vi "CRYTable Empty Ignore.vi"(11 "Table In":string[][](array[string])) -> (3 "Table Out":string[][](array[string]))   [LabVIEW 2013]
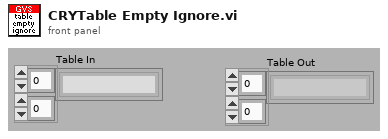
[diagram p1: front panel]
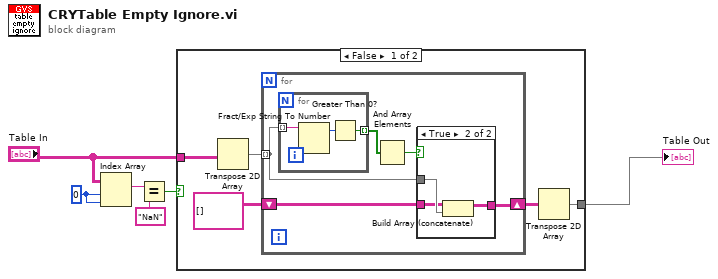
[diagram p0: block diagram]
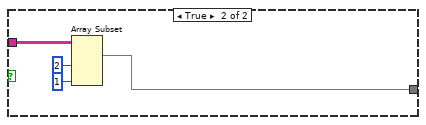
[diagram p3: hidden frame]
diagram:
  w6 = 0 ("Index")
  n1 = Index Array(array="Table In", index (row)=w6, index (col)=w6) -> (element=w5:string)
  n2 = Equal?(x=w5, y="NaN") -> (x = y?=w3:bool)
  n3 = case shown="False" w3 {
    tunnel: "Table In" -> [w11 w25]
    tunnel: [w7 w24] -> w1
    frame False {
      n4 = Transpose 2D Array(2D array=w11) -> (transposed array=w10:string[][])
      n5 = for {
        shift-right: [w16] -> w8
        shift-left: string[][] [] -> [w15]
        tunnel: w10 -> [w13] mode=indexing
        n6 = for {
          tunnel: w13 -> [w19] mode=indexing
          tunnel: [w17] -> w12 mode=indexing
          n7 = Fract/Exp String To Number(string=w19) -> (offset past number=w18:i32)  [unwired: 4 out]
          n8 = Greater Than 0?(x=w18) -> (x > 0?=w17:bool)
        }
        n9 = And Array Elements(Boolean array=w12) -> (logical AND=w14:bool)
        n10 = case shown="True" w14 {
          tunnel: w13 -> [_ w23]
          tunnel: [w20 w22] -> w16
          tunnel: w15 -> [w20 w21]
          frame False {
          }
          frame True {
            n11 = Build Array (concatenate)(w21, w23) -> (w22:string[][])
          }
        }
      }
      n12 = Transpose 2D Array(2D array=w8) -> (transposed array=w7:string[][])
    }
    frame True {
      n13 = Array Subset(array=w25, length (row)=2 ("Array Length"), length (col)=1 ("Array Length")) -> (w24:string[][])  [unwired: 2 in]
    }
  }
  "Table Out" <- w1
